vi "In Range Logic.vi"(9 "Arm Motor":dbl, 10 "Arm Current":dbl, 11 "Arm Set":dbl) -> (3 "In Range":bool)   [LabVIEW 2012]
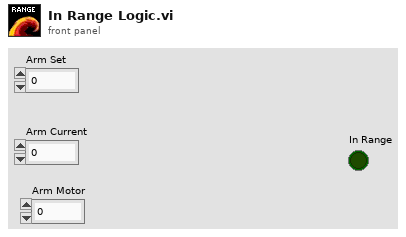
[diagram p1: front panel]
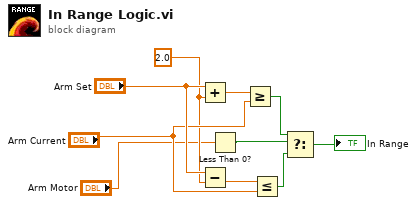
[diagram p0: block diagram]
diagram:
  w3 = 2.0
  n1 = Add(x="Arm Set", y=w3) -> (x+y=w8:dbl)
  n2 = Subtract(x="Arm Set", y=w3) -> (x-y=w9:dbl)
  n3 = Less Than 0?(x="Arm Motor") -> (x < 0?=w2:bool)
  n4 = Greater Or Equal?(x=w8, y="Arm Current") -> (x >= y?=w5:bool)
  n5 = Less Or Equal?(x=w9, y="Arm Current") -> (x <= y?=w6:bool)
  n6 = Select(t=w5, s=w2, f=w6) -> (s? t:f=→"In Range":bool)
